vi "LVCAM Nest Destroyed.vi"(9 "Nest Error":errorcluster, 10 "Nest Actor":refnum<class "LVCAM.lvclass">, 11 "Actor in":refnum<class "Actor.lvclass">) -> (0 "error out":errorcluster, 3 "Actor out":refnum<class "Actor.lvclass">)   [LabVIEW 2021, in "LVCAM.lvlib" / "Actor.lvclass"]
uses:
  Actor.lvclass
  C:/PPLs/LabVIEW-Composed-Actor-Model-LVCAM/LabVIEW-Composed-Actor-Model-LVCAM/LVCAM/LVCAM/LVCAM/LVCAM.lvclass
  LVCAM/LVCAM.lvclass
  Actor.lvclass/Actor.ctl
  Msgs/LVCAM Destroy Self/LVCAM Destroy Self Msg/LVCAM Destroy Self Msg.lvclass
  C:/PPLs/LabVIEW-Composed-Actor-Model-LVCAM/LabVIEW-Composed-Actor-Model-LVCAM/LVCAM/LVCAM/Msg/Msg.lvclass
  Self Msg Send.vi
  C:/PPLs/LabVIEW-Composed-Actor-Model-LVCAM/LabVIEW-Composed-Actor-Model-LVCAM/LVCAM/Msgs/LVCAM Create Nest/LVCAM Create Nest/LVCAM Create Nest.lvclass
  C:/PPLs/LabVIEW-Composed-Actor-Model-LVCAM/LabVIEW-Composed-Actor-Model-LVCAM/LVCAM/Msgs/LVCAM Destroy Self/LVCAM Destroy Self/LVCAM Destroy Self.lvclass
  C:/PPLs/LabVIEW-Composed-Actor-Model-LVCAM/LabVIEW-Composed-Actor-Model-LVCAM/LVCAM/Msgs/LVCAM Nest Destroyed/LVCAM Nest Destroyed/LVCAM Nest Destroyed.lvclass
  C:/PPLs/LabVIEW-Composed-Actor-Model-LVCAM/LabVIEW-Composed-Actor-Model-LVCAM/LVCAM/LVCAM/LVCAM Create/LVCAM Create.lvclass
  C:/PPLs/LabVIEW-Composed-Actor-Model-LVCAM/LabVIEW-Composed-Actor-Model-LVCAM/LVCAM/LVCAM/LVCAM Destroy/LVCAM Destroy.lvclass
  C:/PPLs/LabVIEW-Composed-Actor-Model-LVCAM/LabVIEW-Composed-Actor-Model-LVCAM/LVCAM/LVCAM/LVCAM Error/LVCAM Error.lvclass
  C:/PPLs/LabVIEW-Composed-Actor-Model-LVCAM/LabVIEW-Composed-Actor-Model-LVCAM/LVCAM/LVCAM/LVCAM Receive/LVCAM Receive.lvclass
  C:/PPLs/LabVIEW-Composed-Actor-Model-LVCAM/LabVIEW-Composed-Actor-Model-LVCAM/LVCAM/LVCAM/Actor/Actor.lvclass
  C:/PPLs/LabVIEW-Composed-Actor-Model-LVCAM/LabVIEW-Composed-Actor-Model-LVCAM/LVCAM/Msgs/LVCAM Destroy Self/LVCAM Destroy Self Msg/LVCAM Destroy Self Msg.lvclass
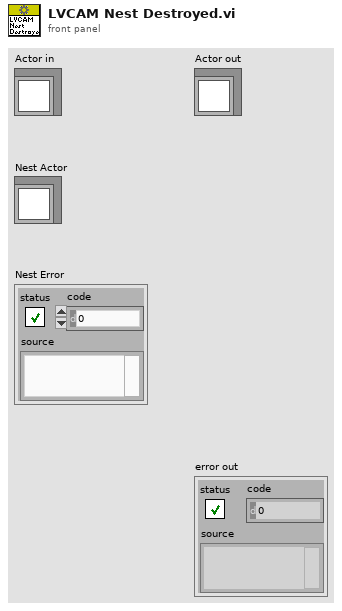
[diagram p1: front panel]
types:
  T1 = typedef "LVCAM.lvlib/Actor.lvclass/State.ctl" = enum16{"Msging", "Destroying"}
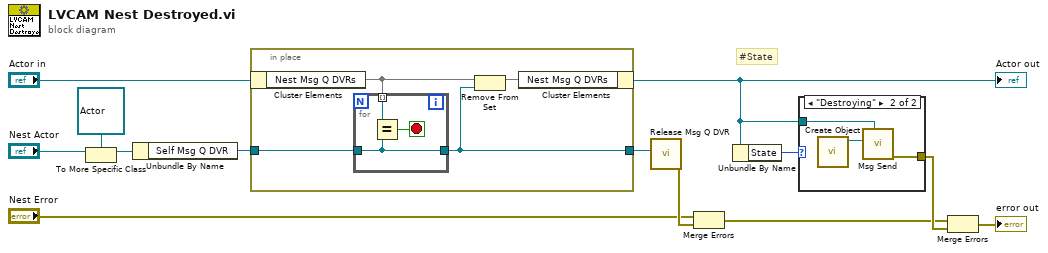
[diagram p0: block diagram]
diagram:
  # "#State"
  n1 = To More Specific Class(target class=refnum<class "Actor.lvclass"> refnum ("Artifex Actor Model.lvlib:Self Actor.lvclass"), reference="Nest Actor") -> (specific class reference=w13:refnum<class "Actor.lvclass">)  [unwired: 1 in, 1 out]
  n2 = Unbundle By Name(w13) -> ("Self Msg Q DVR"=w6:refnum<data-value>)
  n3 = in-place {
    in-place-border: w6 -> [w15]
    in-place-border: [w14] -> w4
    n4 = in-place-cluster #1("Actor in") -> ("Nest Msg Q DVRs"=w17:set{refnum<data-value>})
    n5 = for {
      tunnel: w15 -> [w18]
      tunnel: w17 -> [w19] mode=indexing
      tunnel: [w18] -> w14
      stop <- w20 stop-if-true
      n6 = Equal?(x=w19, y=w18) -> (x = y?=w20:bool)
    }
    n7 = Remove From Set(10:w14, 11:w17) -> (3:w16:set{refnum<data-value>})  [unwired: 1 out]
    n8 = in-place-cluster #1("Nest Msg Q DVRs"=w16) -> (w5:refnum<class "Actor.lvclass">)
  }
  "Actor out" <- w5
  n9 = call "Release Msg Q DVR.vi"("Msg Q DVR"=w4) -> ("error out"=w2:errorcluster)  [unwired: 10 in]
  n10 = Merge Errors("Nest Error", w2) -> (w3:errorcluster)
  n11 = Unbundle By Name(w5) -> ("State"=w9:T1)
  n12 = case shown="\"Destroying\"" w9 {
    tunnel: w5 -> [_ w23]
    tunnel: [_ w21] -> w7
    frame "Msging" {
    }
    frame "Destroying" {
      n13 = call "Create Object.vi"() -> ("LVCAM Destroy Self Msg out"=w22:refnum<class "LVCAM Destroy Self Msg.lvclass">)  [unwired: 11 in]
      n14 = call-poly "Msg Send.vi"("Actor"=w23, "Msg"=w22) -> ("error out"=w21:errorcluster)  [unwired: 9 in]
    }
  }
  n15 = Merge Errors(w3, w7) -> (→"error out":errorcluster)
